vi "AutoZero Driver.vi"(8 "error in (no error)":errorcluster, 10 "AutoZero VSEC":dbl format="%#_13g", 11 "Cree Comms in":refnum<class "Cree Communications.lvclass">) -> (0 "error out":errorcluster)   [LabVIEW 2015, in "Calibration.lvclass"]
uses:
  Calibration.lvclass
  Classes/Cree Communications/Class/Cree Communications.lvclass
  Classes/Cree Communications/Cree Comms Messages/Set AutoZero Calibration/Set AutoZero Calibration.lvclass
  Classes/Cree Communications/Cree Comms Messages/Set Vsec/Set Vsec Reference.lvclass
  Classes/Cree Communications/Cree Comms Messages/CC Message/CC Message.lvclass
  Classes/Cree Communications/Cree Comms Messages/Get AutoZero State/Get AutoZero State.lvclass
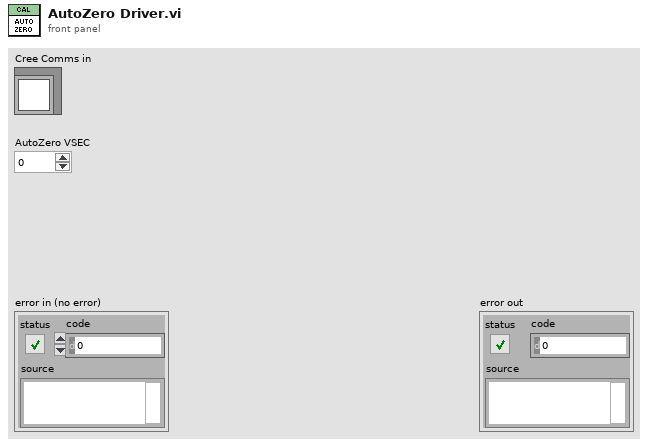
[diagram p1: front panel]
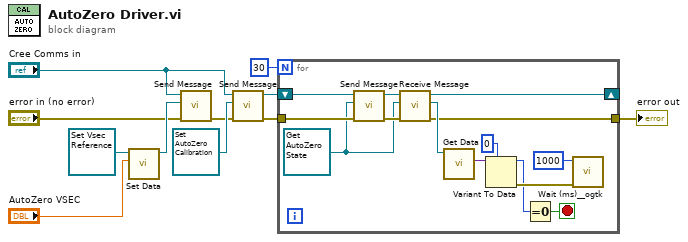
[diagram p0: block diagram]
diagram:
  n1 = call "Set Data.vi"("Data"="AutoZero VSEC", "CC Message in"=refnum<class "Set Vsec Reference.lvclass"> refnum ("Cree Comms Messages.lvlib:Set Vsec Reference.lvclass")) -> ("CC Message out"=w5:refnum<class "Set Vsec Reference.lvclass">)  [unwired: 8 in, 1 out]
  n2 = call "Send Message.vi"("error in (no error)"="error in (no error)", "Cree Comms Message"=w5, "Acrobat Template in"="Cree Comms in") -> ("error out"=w6:errorcluster)  [unwired: 7 in, 1 out]
  n3 = call "Send Message.vi"("error in (no error)"=w6, "Cree Comms Message"=refnum<class "Set AutoZero Calibration.lvclass"> refnum ("Cree Comms Messages.lvlib:Set AutoZero Calibration.lvclass"), "Acrobat Template in"="Cree Comms in") -> ("error out"=w10:errorcluster, "Acrobat Template out"=w9:refnum<class "Cree Communications.lvclass">)  [unwired: 7 in]
  n4 = for {
    N: 30 -> [_]
    tunnel: w10 -> [w24]
    shift-right: [w12] -> _
    shift-left: w9 -> [w25]
    tunnel: [w13] -> w1
    stop <- w14 stop-if-true
    w19 = refnum<class "Get AutoZero State.lvclass"> refnum ("Cree Comms Messages.lvlib:Get AutoZero State.lvclass")
    n5 = call "Send Message.vi"("error in (no error)"=w24, "Cree Comms Message"=w19, "Acrobat Template in"=w25) -> ("error out"=w22:errorcluster, "Acrobat Template out"=w23:refnum<class "Cree Communications.lvclass">)  [unwired: 7 in]
    n6 = call "Receive Message.vi"("error in (no error)"=w22, "CC Message"=w19, "Acrobat Template in"=w23) -> ("error out"=w13:errorcluster, "Cree Comms Message"=w21:refnum<class "CC Message.lvclass">, "Acrobat Template out"=w12:refnum<class "Cree Communications.lvclass">)  [unwired: 6 in]
    n7 = call "Get Data.vi"("CC Message in"=w21) -> ("Data"=w20:variant)  [unwired: 8 in, 2 out]
    n8 = Variant To Data(type=u8 0 ("Response Type"), Variant=w20) -> (data=w15:u8, error out=w16:errorcluster)  [unwired: 1 in]
    n9 = Equal To 0?(x=w15) -> (x = 0?=w14:bool)
    n10 = call <userlib>:"Wait (ms)__ogtk.vi"("error in (no error)"=w16, "milliseconds to wait"=u32 1000) -> ()  [unwired: 8 in, 2 out]
  }
  "error out" <- w1
